vi "Write Image.vi"(8 "error in (no error)":errorcluster, 9 "2D Picture":picture, 11 "48x64 I2C OLED SSD1306 In":refnum<class "48x64 I2C OLED SSD1306.lvclass">) -> (0 "error out":errorcluster, 3 "48x64 I2C OLED SSD1306 Out":refnum<class "48x64 I2C OLED SSD1306.lvclass">)   [LabVIEW 2020, in "CTI-Peripheral.lvlib" / "48x64 I2C OLED SSD1306.lvclass"]
uses:
  48x64 I2C OLED SSD1306.lvclass
  48x64 I2C OLED SSD1306.lvclass/48x64 I2C OLED SSD1306.ctl
  CTI/I2C Connection/I2C Connection.lvclass/I2C Connection.ctl
  Private/BuildMessagesFromPicture.vi
  CTI/Session/I2C Write Data.vi
  CTI/I2C Connection/I2C Connection.lvclass
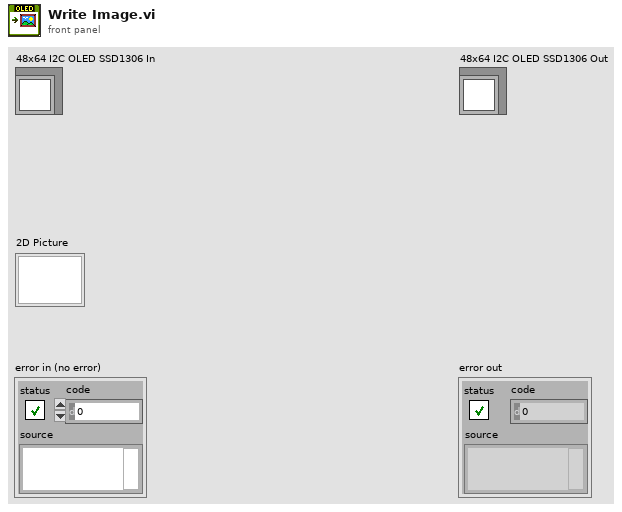
[diagram p1: front panel]
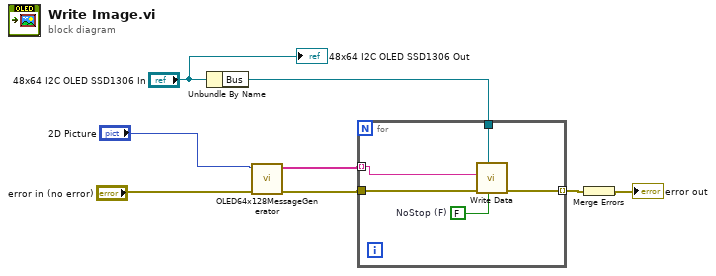
[diagram p0: block diagram]
diagram:
  n1 = Unbundle By Name("48x64 I2C OLED SSD1306 In") -> ("Bus"=w4:refnum<class "I2C Connection.lvclass">)
  n2 = call-poly "OLED64x128MessageGenerator.vi"("error in (no error)"="error in (no error)", "2D Picture"="2D Picture") -> ("error out"=w7:errorcluster, "Messages"=w8:string[])  [unwired: 8 in]
  n3 = for {
    tunnel: w4 -> [w12]
    tunnel: w8 -> [w9] mode=indexing
    tunnel: w7 -> [w10]
    tunnel: [w13] -> w1 mode=indexing
    w11 = FALSE  # NoStop (F)
    n4 = call "Write Data.vi"("NoStop (F)"=w11, "I2C Connection"=w12, "error in (no error)"=w10, "Data"=w9) -> ("error out"=w13:errorcluster)  [unwired: 7 in]
  }
  n5 = Merge Errors(w1) -> (→"error out":errorcluster)
  "48x64 I2C OLED SSD1306 Out" <- "48x64 I2C OLED SSD1306 In"
